vi "MainSockets.vi"() -> ()   [LabVIEW 2018]
uses:
  <vilib>/addons/zeromq/zmq_context.lvclass
  socket REP/socket REP.lvclass
  C:/Users/Denis/Desktop/communication-manager/communication-manager/Socket/Socket.lvclass
  socket REQ/socket REQ.lvclass
  socket SUB/socket SUB.lvclass
  socket PUB/socket PUB.lvclass
  RxTx/RxTx.lvclass
  Socket/Socket.lvclass
panel:
  in  "socket PUB.lvclass":refnum<class "socket PUB.lvclass">
  in  "socket SUB.lvclass":refnum<class "socket SUB.lvclass">
  in  "socket REQ.lvclass":refnum<class "socket REQ.lvclass">
  in  "socket REP.lvclass":refnum<class "socket REP.lvclass">
  out "context":refnum<class "zmq_context.lvclass">
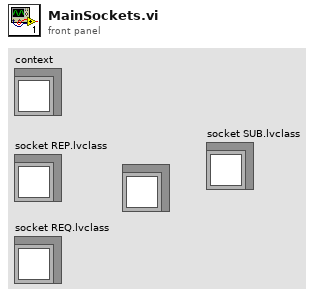
[diagram p1: front panel]
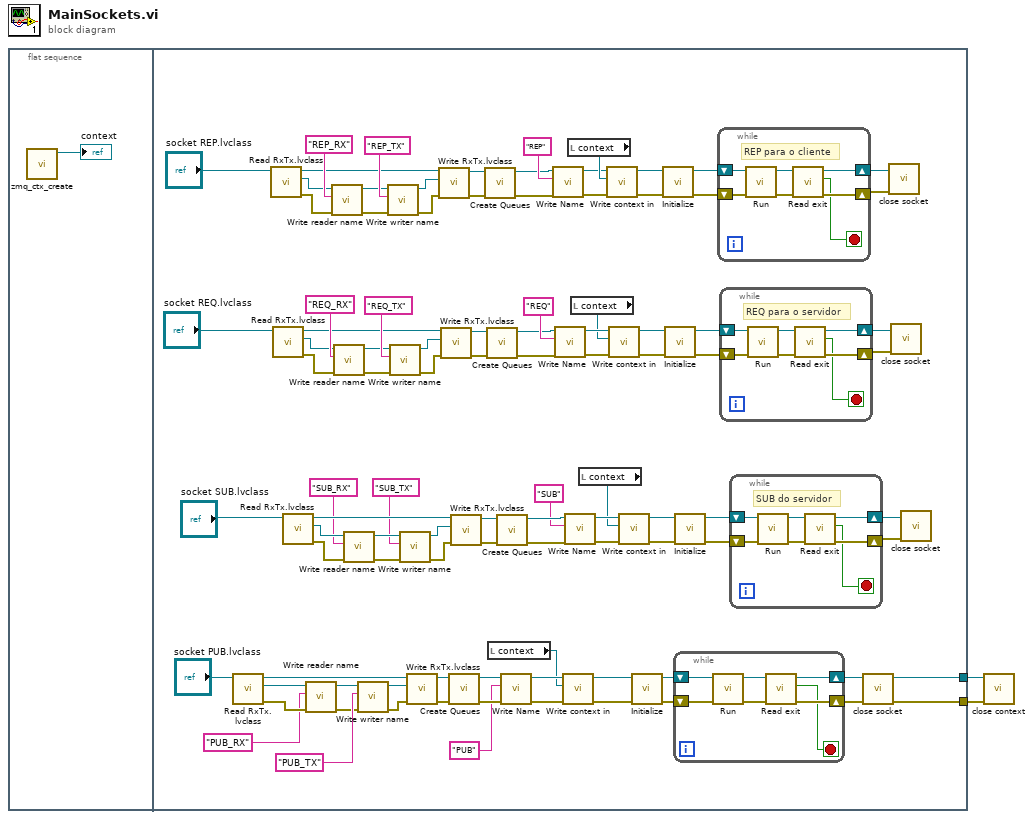
[diagram p0: block diagram]
diagram:
  n1 = flat-sequence {
    tunnel: [w5] -> w2
    tunnel: [w4] -> w1
    frame #0 {
      n2 = call <vilib>:"zmq_ctx_create.vi"() -> ("context out"=→"context":refnum<class "zmq_context.lvclass">)  [unwired: 4 in, 1 out]
    }
    frame #1 {
      n3 = call-dynamic "Read RxTx.lvclass.vi"("Socket in"="socket PUB.lvclass") -> ("error out"=w94:errorcluster, "RxTx.lvclass"=w100:refnum<class "RxTx.lvclass">, "Socket out"=w97:refnum<class "socket PUB.lvclass">)  [unwired: 8 in]
      n4 = call-dynamic "Read RxTx.lvclass.vi"("Socket in"="socket REP.lvclass") -> ("error out"=w21:errorcluster, "RxTx.lvclass"=w27:refnum<class "RxTx.lvclass">, "Socket out"=w24:refnum<class "socket REP.lvclass">)  [unwired: 8 in]
      n5 = call-dynamic "Read RxTx.lvclass.vi"("Socket in"="socket REQ.lvclass") -> ("error out"=w45:errorcluster, "RxTx.lvclass"=w51:refnum<class "RxTx.lvclass">, "Socket out"=w48:refnum<class "socket REQ.lvclass">)  [unwired: 8 in]
      n6 = call-dynamic "Read RxTx.lvclass.vi"("Socket in"="socket SUB.lvclass") -> ("error out"=w66:errorcluster, "RxTx.lvclass"=w60:refnum<class "RxTx.lvclass">, "Socket out"=w63:refnum<class "socket SUB.lvclass">)  [unwired: 8 in]
      n7 = call-dynamic "Write reader name.vi"("error in (no error)"=w94, "RX name"="PUB_RX" ("reader name"), "RxTx in"=w100) -> ("error out"=w93:errorcluster, "RxTx out"=w99:refnum<class "RxTx.lvclass">)  [unwired: 7 in]
      n8 = call-dynamic "Write reader name.vi"("error in (no error)"=w21, "RX name"="REP_RX" ("reader name"), "RxTx in"=w27) -> ("error out"=w20:errorcluster, "RxTx out"=w26:refnum<class "RxTx.lvclass">)  [unwired: 7 in]
      n9 = call-dynamic "Write reader name.vi"("error in (no error)"=w45, "RX name"="REQ_RX" ("reader name"), "RxTx in"=w51) -> ("error out"=w44:errorcluster, "RxTx out"=w50:refnum<class "RxTx.lvclass">)  [unwired: 7 in]
      n10 = call-dynamic "Write reader name.vi"("error in (no error)"=w66, "RX name"="SUB_RX" ("reader name"), "RxTx in"=w60) -> ("error out"=w67:errorcluster, "RxTx out"=w61:refnum<class "RxTx.lvclass">)  [unwired: 7 in]
      n11 = call-dynamic "Write writer name.vi"("error in (no error)"=w93, "Tx name"="PUB_TX" ("writer name"), "RxTx in"=w99) -> ("error out"=w92:errorcluster, "RxTx out"=w98:refnum<class "RxTx.lvclass">)  [unwired: 7 in]
      n12 = call-dynamic "Write writer name.vi"("error in (no error)"=w20, "Tx name"="REP_TX" ("writer name"), "RxTx in"=w26) -> ("error out"=w19:errorcluster, "RxTx out"=w25:refnum<class "RxTx.lvclass">)  [unwired: 7 in]
      n13 = call-dynamic "Write writer name.vi"("error in (no error)"=w44, "Tx name"="REQ_TX" ("writer name"), "RxTx in"=w50) -> ("error out"=w43:errorcluster, "RxTx out"=w49:refnum<class "RxTx.lvclass">)  [unwired: 7 in]
      n14 = call-dynamic "Write writer name.vi"("error in (no error)"=w67, "Tx name"="SUB_TX" ("writer name"), "RxTx in"=w61) -> ("error out"=w68:errorcluster, "RxTx out"=w62:refnum<class "RxTx.lvclass">)  [unwired: 7 in]
      n15 = call-dynamic "Write RxTx.lvclass.vi"("error in (no error)"=w92, "RxTx.lvclass"=w98, "Socket in"=w97) -> ("error out"=w95:errorcluster, "Socket out"=w96:refnum<class "socket PUB.lvclass">)  [unwired: 7 in]
      n16 = call-dynamic "Write RxTx.lvclass.vi"("error in (no error)"=w19, "RxTx.lvclass"=w25, "Socket in"=w24) -> ("error out"=w22:errorcluster, "Socket out"=w23:refnum<class "socket REP.lvclass">)  [unwired: 7 in]
      n17 = call-dynamic "Write RxTx.lvclass.vi"("error in (no error)"=w43, "RxTx.lvclass"=w49, "Socket in"=w48) -> ("error out"=w46:errorcluster, "Socket out"=w47:refnum<class "socket REQ.lvclass">)  [unwired: 7 in]
      n18 = call-dynamic "Create Queues.vi"("error in (no error)"=w95, "Socket in"=w96) -> ("error out"=w88:errorcluster, "Socket out"=w91:refnum<class "socket PUB.lvclass">)  [unwired: 8 in]
      n19 = call-dynamic "Write RxTx.lvclass.vi"("error in (no error)"=w68, "RxTx.lvclass"=w62, "Socket in"=w63) -> ("error out"=w65:errorcluster, "Socket out"=w64:refnum<class "socket SUB.lvclass">)  [unwired: 7 in]
      n20 = call-dynamic "Create Queues.vi"("error in (no error)"=w22, "Socket in"=w23) -> ("error out"=w12:errorcluster, "Socket out"=w15:refnum<class "socket REP.lvclass">)  [unwired: 8 in]
      n21 = call-dynamic "Create Queues.vi"("error in (no error)"=w46, "Socket in"=w47) -> ("error out"=w38:errorcluster, "Socket out"=w41:refnum<class "socket REQ.lvclass">)  [unwired: 8 in]
      n22 = local read "context"() -> (w80:refnum<class "zmq_context.lvclass">)
      n23 = call-dynamic "Create Queues.vi"("error in (no error)"=w65, "Socket in"=w64) -> ("error out"=w73:errorcluster, "Socket out"=w70:refnum<class "socket SUB.lvclass">)  [unwired: 8 in]
      n24 = call-dynamic "Write Name.vi"("error in (no error)"=w88, "Name"="PUB", "Socket in"=w91) -> ("error out"=w87:errorcluster, "Socket out"=w90:refnum<class "socket PUB.lvclass">)  [unwired: 7 in]
      n25 = call-dynamic "Write Name.vi"("error in (no error)"=w12, "Name"="REP", "Socket in"=w15) -> ("error out"=w11:errorcluster, "Socket out"=w14:refnum<class "socket REP.lvclass">)  [unwired: 7 in]
      n26 = call-dynamic "Write Name.vi"("error in (no error)"=w38, "Name"="REQ", "Socket in"=w41) -> ("error out"=w37:errorcluster, "Socket out"=w40:refnum<class "socket REQ.lvclass">)  [unwired: 7 in]
      n27 = call-dynamic "Write context in.vi"("error in (no error)"=w87, "zeromq.lvlib:ZeroMQ Context"=w80, "Socket in"=w90) -> ("error out"=w86:errorcluster, "Socket out"=w89:refnum<class "socket PUB.lvclass">)  [unwired: 7 in]
      n28 = call-dynamic "Write Name.vi"("error in (no error)"=w73, "Name"="SUB", "Socket in"=w70) -> ("error out"=w74:errorcluster, "Socket out"=w71:refnum<class "socket SUB.lvclass">)  [unwired: 7 in]
      n29 = local read "context"() -> (w16:refnum<class "zmq_context.lvclass">)
      n30 = local read "context"() -> (w30:refnum<class "zmq_context.lvclass">)
      n31 = local read "context"() -> (w57:refnum<class "zmq_context.lvclass">)
      n32 = call-dynamic "Write context in.vi"("error in (no error)"=w11, "zeromq.lvlib:ZeroMQ Context"=w16, "Socket in"=w14) -> ("error out"=w10:errorcluster, "Socket out"=w13:refnum<class "socket REP.lvclass">)  [unwired: 7 in]
      n33 = call-dynamic "Write context in.vi"("error in (no error)"=w37, "zeromq.lvlib:ZeroMQ Context"=w30, "Socket in"=w40) -> ("error out"=w36:errorcluster, "Socket out"=w39:refnum<class "socket REQ.lvclass">)  [unwired: 7 in]
      n34 = call-dynamic "Write context in.vi"("error in (no error)"=w74, "zeromq.lvlib:ZeroMQ Context"=w57, "Socket in"=w71) -> ("error out"=w75:errorcluster, "Socket out"=w72:refnum<class "socket SUB.lvclass">)  [unwired: 7 in]
      n35 = call-dynamic "Initialize.vi"("error in (no error)"=w86, "socket PUB in"=w89) -> ("error out"=w83:errorcluster, "socket PUB out"=w85:refnum<class "socket PUB.lvclass">)  [unwired: 8 in]
      n36 = call-dynamic "Initialize.vi"("error in (no error)"=w10, "socket REP in"=w13) -> ("error out"=w7:errorcluster, "socket REP out"=w9:refnum<class "socket REP.lvclass">)  [unwired: 8 in]
      n37 = call-dynamic "Initialize.vi"("error in (no error)"=w36, "socket REQ in"=w39) -> ("error out"=w33:errorcluster, "socket REQ out"=w35:refnum<class "socket REQ.lvclass">)  [unwired: 8 in]
      n38 = while {
        shift-right: [w125] -> w84
        shift-left: w85 -> [w129]
        shift-right: [w124] -> w82
        shift-left: w83 -> [w128]
        stop <- w123 stop-if-true
        n39 = call-dynamic "Run.vi"("error in (no error)"=w128, "socket PUB in"=w129) -> ("error out"=w127:errorcluster, "socket PUB out"=w126:refnum<class "socket PUB.lvclass">)  [unwired: 8 in]
        n40 = call-dynamic "Read exit.vi"("error in (no error)"=w127, "Socket in"=w126) -> ("error out"=w124:errorcluster, "exit"=w123:bool, "Socket out"=w125:refnum<class "socket PUB.lvclass">)  [unwired: 7 in]
      }
      n41 = call-dynamic "Initialize.vi"("error in (no error)"=w75, "socket SUB in"=w72) -> ("error out"=w78:errorcluster, "socket SUB out"=w76:refnum<class "socket SUB.lvclass">)  [unwired: 8 in]
      n42 = while {
        shift-right: [w106] -> w8
        shift-left: w9 -> [w108]
        shift-right: [w103] -> w6
        shift-left: w7 -> [w105]
        stop <- w102 stop-if-true
        # "REP para o cliente"
        n43 = call-dynamic "Run.vi"("error in (no error)"=w105, "socket REP in"=w108) -> ("error out"=w104:errorcluster, "socket REP out"=w107:refnum<class "socket REP.lvclass">)  [unwired: 8 in]
        n44 = call-dynamic "Read exit.vi"("error in (no error)"=w104, "Socket in"=w107) -> ("error out"=w103:errorcluster, "exit"=w102:bool, "Socket out"=w106:refnum<class "socket REP.lvclass">)  [unwired: 7 in]
      }
      n45 = while {
        shift-right: [w113] -> w34
        shift-left: w35 -> [w115]
        shift-right: [w110] -> w32
        shift-left: w33 -> [w112]
        stop <- w109 stop-if-true
        # "REQ para o servidor"
        n46 = call-dynamic "Run.vi"("error in (no error)"=w112, "socket REQ in"=w115) -> ("error out"=w111:errorcluster, "socket REQ out"=w114:refnum<class "socket REQ.lvclass">)  [unwired: 8 in]
        n47 = call-dynamic "Read exit.vi"("error in (no error)"=w111, "Socket in"=w114) -> ("error out"=w110:errorcluster, "exit"=w109:bool, "Socket out"=w113:refnum<class "socket REQ.lvclass">)  [unwired: 7 in]
      }
      n48 = while {
        shift-right: [w120] -> w77
        shift-left: w76 -> [w122]
        shift-right: [w117] -> w79
        shift-left: w78 -> [w119]
        stop <- w116 stop-if-true
        # "SUB do servidor"
        n49 = call-dynamic "Run.vi"("error in (no error)"=w119, "socket SUB in"=w122) -> ("error out"=w118:errorcluster, "socket SUB out"=w121:refnum<class "socket SUB.lvclass">)  [unwired: 8 in]
        n50 = call-dynamic "Read exit.vi"("error in (no error)"=w118, "Socket in"=w121) -> ("error out"=w117:errorcluster, "exit"=w116:bool, "Socket out"=w120:refnum<class "socket SUB.lvclass">)  [unwired: 7 in]
      }
      n51 = call "close socket.vi"("error in (no error)"=w82, "Socket in"=w84) -> ("error out"=w5:errorcluster, "Socket out"=w4:refnum<class "socket PUB.lvclass">)  [unwired: 8 in]
      n52 = call "close socket.vi"("error in (no error)"=w6, "Socket in"=w8) -> ()  [unwired: 8 in, 2 out]
      n53 = call "close socket.vi"("error in (no error)"=w32, "Socket in"=w34) -> ()  [unwired: 8 in, 2 out]
      n54 = call "close socket.vi"("error in (no error)"=w79, "Socket in"=w77) -> ()  [unwired: 8 in, 2 out]
    }
  }
  n55 = call-dynamic "close context.vi"("error in (no error)"=w2, "Socket in"=w1) -> ()  [unwired: 8 in, 2 out]
